vi "Set Params.vi"(6 "Lengths.a 2":dbl, 7 "Lengths.a 3":dbl, 8 "error in (no error)":errorcluster, 9 "Lengths.a":dbl, 10 "CoordinatesIN":cluster{"X":dbl, "Y":dbl, "Z":dbl}, 11 "reference in":refnum<class "Manipulator.lvclass">) -> (0 "error out":errorcluster, 3 "reference out":refnum<class "Manipulator.lvclass">)   [LabVIEW 2014, in "Manipulator.lvclass"]
uses:
  Manipulator.lvclass
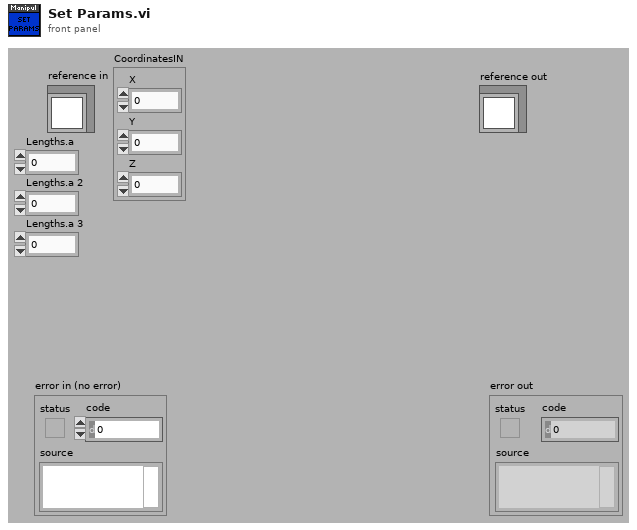
[diagram p1: front panel]
types:
  T1 = typedef "Manipulator.lvclass/ObjectAttributes.ctl" = cluster{"Coordinates":cluster{"X":dbl, "Y":dbl, "Z":dbl}, "Angles":cluster{"THETA_1":dbl, "THETA_2":dbl, "THETA_3":dbl, "THETA_4":dbl, "THETA_5":dbl, "THETA_6":dbl, "THETA_7":dbl, "THETA_8":dbl, "THETA_9":dbl, "THETA_10":dbl}, "Lengths":cluster{"a":dbl, "b":dbl, "c":dbl, "d":dbl, "e":dbl}}
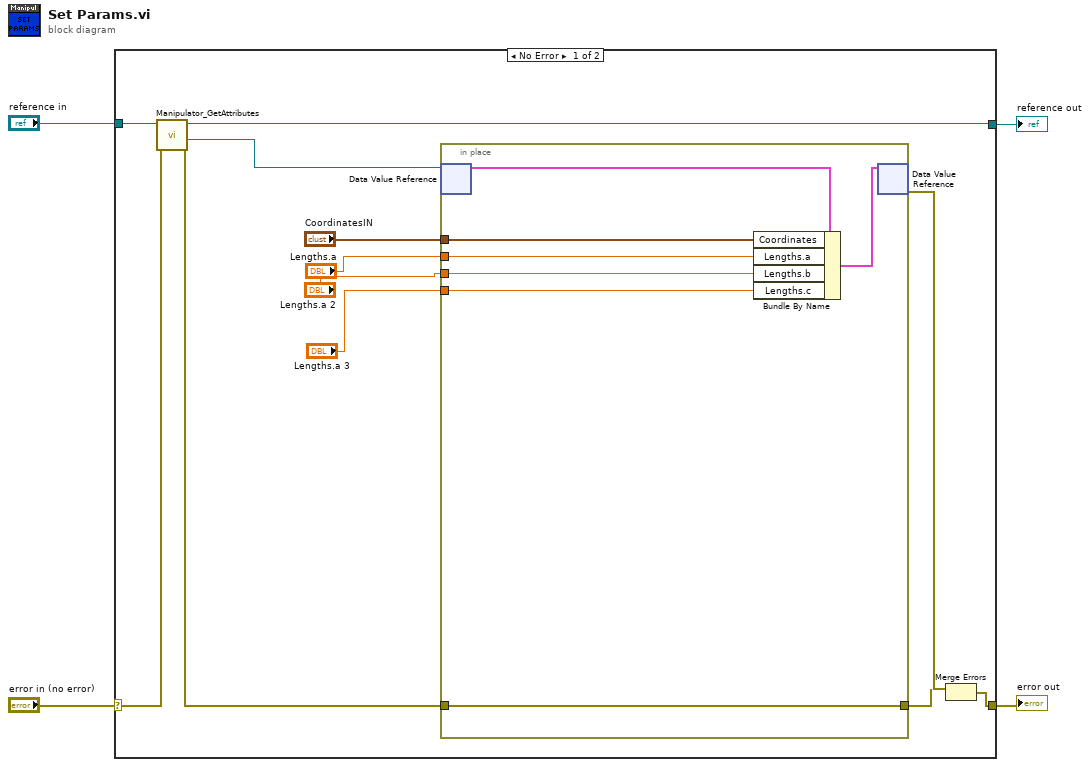
[diagram p0: block diagram]
diagram:
  n1 = case shown="No Error" "error in (no error)" {
    selector: "error in (no error)" -> [w15 w25]
    tunnel: [w12 w25] -> w3
    tunnel: [w13 w24] -> w1
    tunnel: "reference in" -> [w16 w24]
    frame No Error {
      n2 = call "Manipulator_GetAttributes.vi"("error in (no error)"=w15, "reference in"=w16) -> ("error out"=w10:errorcluster, "DataRef"=w11:refnum<data-value>, "reference out"=w13:refnum<class "Manipulator.lvclass">)  [unwired: 6 in, 1 out]
      n3 = in-place {
        in-place-border: w10 -> [w23]
        in-place-border: [w23] -> w9
        in-place-border: "CoordinatesIN" -> [w21]
        in-place-border: "Lengths.a" -> [w19]
        in-place-border: "Lengths.a 2" -> [w18]
        in-place-border: "Lengths.a 3" -> [w17]
        n4 = in-place-dvr #1(w11) -> (w22:T1)  [unwired: 1 out]
        n5 = Bundle By Name(cluster=w22, "Coordinates"=w21, "Lengths.a"=w19, "Lengths.b"=w18, "Lengths.c"=w17) -> (w20:T1)
        n6 = in-place-dvr #1(w20) -> (w14:errorcluster)  [unwired: 1 out]
      }
      n7 = Merge Errors(w14, w9) -> (w12:errorcluster)
    }
    frame Error {
    }
  }
  "error out" <- w3
  "reference out" <- w1
